vi "rs3 Advanced set depth control3.vi"(8 "error in (no error)":errorcluster, 10 "depth control":T1, 11 "device in":u64) -> (0 "error out":errorcluster, 1 "error":u64, 3 "Dev out":u64)   [LabVIEW 2019, in "libRealSense3.lvlib"]
doc: "Sets registers inside the ASIC that affect the depth calculations"
uses:
  libRealSense3.lvlib
  realsense2.dll
panel:
  # "RS3 Adv. Set Depth Control 2"
  # "(C) 2017 Intel Corp.,  AGJ"
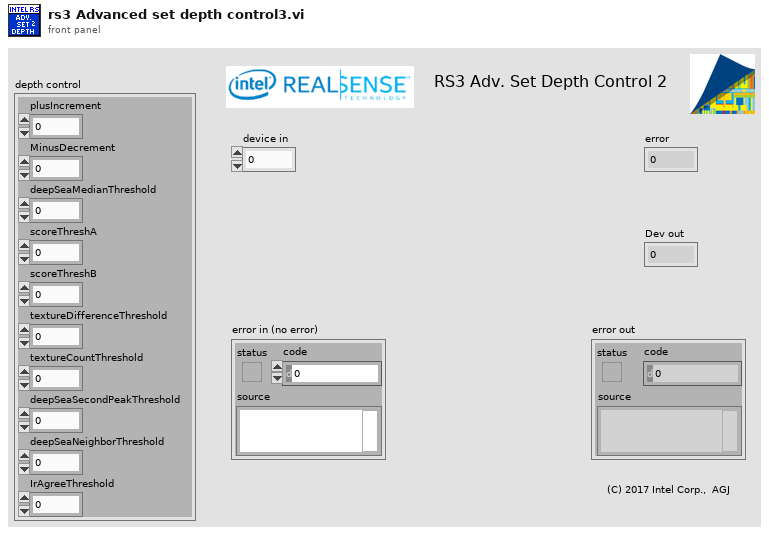
[diagram p1: front panel]
types:
  T1 = cluster{"plusIncrement":u32, "MinusDecrement":u32, "deepSeaMedianThreshold":u32, "scoreThreshA":u32, "scoreThreshB":u32, "textureDifferenceThreshold":u32, "textureCountThreshold":u32, "deepSeaSecondPeakThreshold":u32, "deepSeaNeighborThreshold":u32, "IrAgreeThreshold":u32}
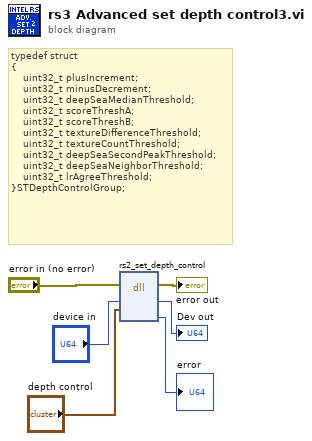
[diagram p0: block diagram]
diagram:
  # "typedef struct\n{\n    uint32_t plusIncrement;\n    uint32_t minusDecrement;\n    uint32_t deepSeaMedianThreshold;\n    uint32_t scoreThreshA;\n    uint32_t scoreThreshB;\n    uint32_t textureDifferenceThreshold;\n    uint32_t textureCountThreshold;\n    uint32_t deepSeaSecondPeakThreshold;\n    uint32_t deepSeaNeighborThreshold;\n    uint32_t lrAgreeThreshold;\n}STDepthControlGroup;"
  n1 = dll-call lib="C:/Users/morte/Documents/gitmoro/treadmill/RealSense for Labview ver. 2.33/realsense2.dll" fn="rs2_set_depth_control"(error in="error in (no error)", "device"="device in", "depth control"="depth control") -> (error out=→"error out":errorcluster, "device"=→"Dev out":u64, "error"=→"error":u64)  [unwired: 5 in, 1 out]
